vi "CRYReplace Name From Step.vi"(9 "New Name":string, 10 "Old Name":string, 11 "Type In":enum16{"Curves", "Values", "Results", "WFM"}(ring)) -> (2 "Replaced Name Out":string, 3 "No Name?":bool)   [LabVIEW 2013]
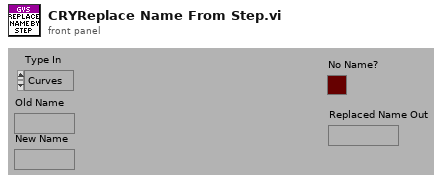
[diagram p1: front panel]
types:
  T1 = typedef "CRYData Cluster.ctl" = cluster{"Name":string, "Curve":cluster{"x":dbl, "y":dbl, "z":dbl}[], "X data":u16, "Y data":u16, "Z data":u16, "X axis":u16, "Y axis":u16, "Z axis":u16, "X unit":string, "Y unit":string, "Z unit":string, "X dB ref":dbl, "Y dB ref":dbl, "Z dB ref":dbl, "single val":bool, "protected":bool, "display X":bool, "display Y":bool, "display Z":bool, "Test Info":string, "Step No.":i32, "Plot Settings":cluster{"Color":u32, "Interpolation":u8, "Point Style":u8, "Line Style":u8, "Point Color":u32, "Line Width":u8, "Bar Plot Style":u8, "Fill To":i16}, "AutoProtect":bool}
  T2 = typedef "CRYWaveform Cluster.ctl" = cluster{"Waveform":cluster{"X0":dbl, "dX":dbl, "Y":sgl[]}, "X data":u16, "Y data":u16, "Y axis":u16, "X unit":string, "Y unit":string, "Y dB ref":dbl, "display Y":bool, "display X":bool, "Overload?":bool, "Test Info":string, "Step No.":i32, "Name":string, "protected":bool, "Sqc history":string[], "Signal Channel ID":i32, "Plot Settings":cluster{"Color":u32, "Interpolation":u8, "Point Style":u8, "Line Style":u8, "Point Color":u32, "Line Width":u8, "Bar Plot Style":u8, "Fill To":i16}, "AutoProtect":bool}
  T3 = typedef "CRYResult Cluster.ctl" = cluster{"Name":string, "Margin":dbl, "unit":string, "Verdict":bool, "Limit":string, "Max/Min":string, "protected":bool, "Step No.":i32, "Test Info":string, "AutoProtect":bool}
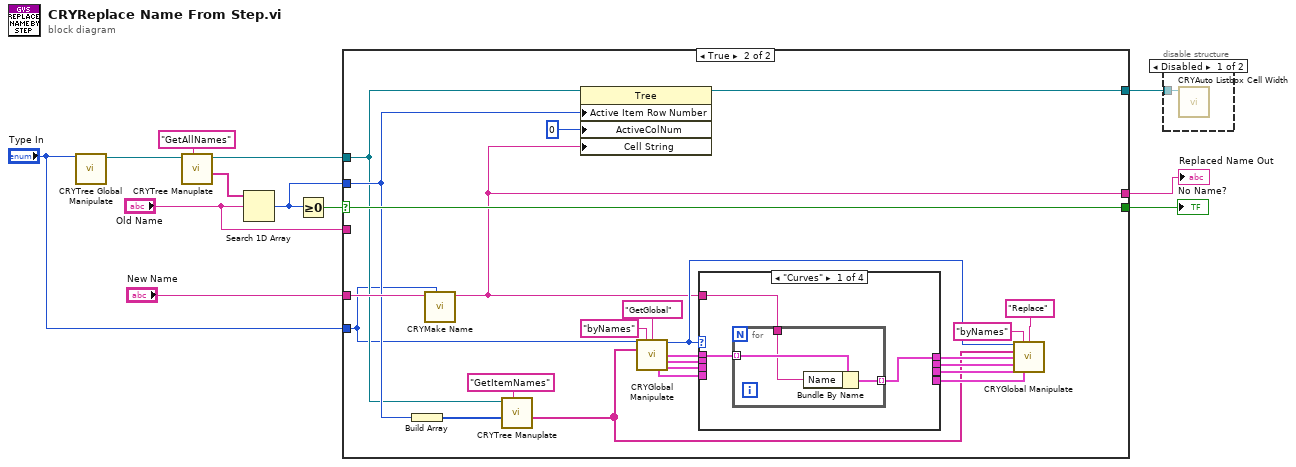
[diagram p0: block diagram]
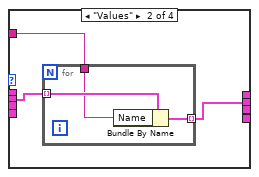
[diagram p4: hidden frame]
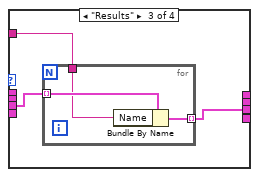
[diagram p5: hidden frame]
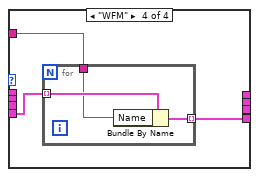
[diagram p6: hidden frame]
diagram:
  n1 = call "CRYTree Global Manipulate.vi"("Type In"="Type In") -> ("Tree/Curve Tree"=w3:refnum<vi>)  [unwired: 7 in, 3 out]
  n2 = call "CRYTree Manuplate.vi"("sAction"="GetAllNames", "Tree in"=w3) -> ("sData Out"=w4:string[], "Tree Out"=w1:refnum<vi>)  [unwired: 6 in, 2 out]
  n3 = Search 1D Array(1D array=w4, element="Old Name") -> (index of element=w10:i32)  [unwired: 1 out]
  n4 = Greater Or Equal To 0?(x=w10) -> (x >= 0?=w11:bool)
  n5 = case shown="True" w11 {
    selector: w11 -> [w15 w39]
    tunnel: [w13 w36] -> w9
    tunnel: w10 -> [_ w23]
    tunnel: "New Name" -> [_ w38]
    tunnel: [w15 w39] -> w8
    tunnel: "Type In" -> [_ w17]
    tunnel: [w14 w22] -> w7
    tunnel: "Old Name" -> [w14 _]
    tunnel: w1 -> [w13 w20]
    frame False {
    }
    frame True {
      n6 = Build Array(w23) -> (w19:i32[])
      n7 = call "CRYMake Name.vi"("Type"=w17, "Name In"=w38) -> ("Name Out"=w22:string)  [unwired: 5 in, 4 out]
      n8 = call "CRYTree Manuplate.vi"("sAction"="GetItemNames", "nData"=w19, "Tree in"=w20) -> ("sData Out"=w18:string[])  [unwired: 5 in, 3 out]
      n9 = property on="Property Node" class="Tree"(reference=w20, "Active Item Row Number"=w23, "ActiveColNum"=0 ("Active Cell:Active Column Number"), "Cell String"=w22) -> (reference out=w36:refnum<vi>)  [unwired: 1 in, 1 out]
      n10 = call "CRYGlobal Manipulate.vi"("Type"=w17, "sOption"="byNames", "sAction"="GetGlobal", "sData"=w18) -> ("Type out"=w30:enum16{"Curves", "Values", "Results", "WFM"}, "Curves Out"=w35:T1[], "Values Out"=w29:T1[], "WFM Out"=w27:T2[], "Results Out"=w28:T3[])  [unwired: 5 in, 2 out]
      n11 = case shown="\"Curves\"" w30 {
        tunnel: w35 -> [w42 _ _ _]
        tunnel: [w41 _ _ _] -> w31
        tunnel: w29 -> [_ w48 _ _]
        tunnel: w28 -> [_ _ w54 _]
        tunnel: w27 -> [_ _ _ w60]
        tunnel: [_ w47 _ _] -> w26
        tunnel: [_ _ w53 _] -> w25
        tunnel: [_ _ _ w59] -> w24
        tunnel: w22 -> [w40 w46 w52 w58]
        frame "Curves" {
          n12 = for {
            tunnel: w42 -> [w44] mode=indexing
            tunnel: [w45] -> w41 mode=indexing
            tunnel: w40 -> [w43]
            n13 = Bundle By Name(cluster=w44, "Name"=w43) -> (w45:T1)
          }
        }
        frame "Values" {
          n14 = for {
            tunnel: w48 -> [w50] mode=indexing
            tunnel: [w51] -> w47 mode=indexing
            tunnel: w46 -> [w49]
            n15 = Bundle By Name(cluster=w50, "Name"=w49) -> (w51:T1)
          }
        }
        frame "Results" {
          n16 = for {
            tunnel: w54 -> [w56] mode=indexing
            tunnel: [w57] -> w53 mode=indexing
            tunnel: w52 -> [w55]
            n17 = Bundle By Name(cluster=w56, "Name"=w55) -> (w57:T3)
          }
        }
        frame "WFM" {
          n18 = for {
            tunnel: w60 -> [w62] mode=indexing
            tunnel: [w63] -> w59 mode=indexing
            tunnel: w58 -> [w61]
            n19 = Bundle By Name(cluster=w62, "Name"=w61) -> (w63:T2)
          }
        }
      }
      n20 = call "CRYGlobal Manipulate.vi"("Type"=w30, "sOption"="byNames", "sAction"="Replace", "sData"=w18, "Curves"=w31, "Values"=w26, "Results"=w25, "WFM"=w24) -> ()  [unwired: 1 in, 7 out]
    }
  }
  "No Name?" <- w8
  "Replaced Name Out" <- w7
  n21 = disable-structure shown="Disabled" {
    disable-tunnel: w9 -> [w64 _]
    frame Disabled {
      n22 = call "CRYAuto Listbox Cell Width.vi"("Listbox In"=w64) -> ()  [unwired: 10 in, 1 out]
    }
    frame Enabled {
    }
  }
